vi "AddFailure_WithParent_ParentFailureIconSet.vi"() -> (0 "error out":errorcluster)   [LabVIEW 2017, in "ResultTreeListenerTest.lvlib"]
uses:
  ResultTreeListenerTest.lvlib
  ResultTreeListener/ResultTreeListener.lvclass
  ResultTree/ResultTree.lvclass
  Support/FakeTestCase/FakeTestCase.lvclass
  C:/Users/de200256/Code/neuperger/lvunit/Test/Test.lvclass
  275d98eb-69a7-4435-8809-2af3ffd1cf1d.vi
  ResultTree/Icon.ctl
  Support/FakeTestSuite/FakeTestSuite.lvclass
  C:/Users/de200256/Code/neuperger/lvunit/TestSuite/TestSuite.lvclass
panel:
  in  "Tree":string(tree)
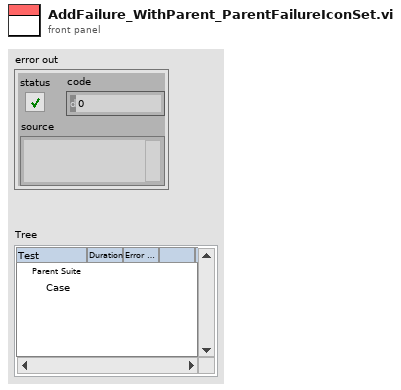
[diagram p1: front panel]
types:
  T1 = typedef "ResultTree.lvclass/Icon.ctl" = enum16{"None", "Passed", "Failed", "Error"}
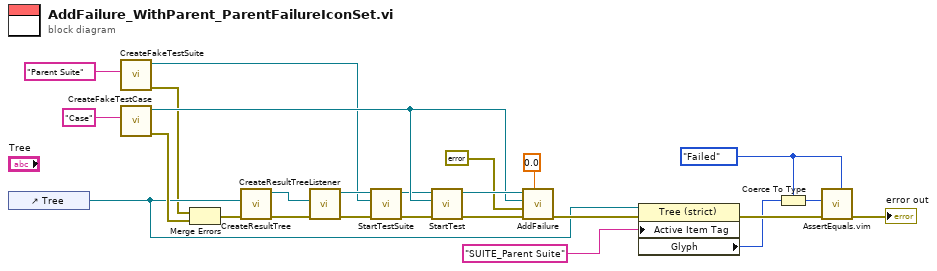
[diagram p0: block diagram]
diagram:
  w8 = Icon."Failed" ("Active Cell:String")
  n1 = control-ref of="Tree"() -> (w13:refnum<vi>)
  n2 = call "CreateFakeTestSuite.vi"("Name"="Parent Suite") -> ("error out"=w5:errorcluster, "FakeTestSuite out"=w1:refnum<class "FakeTestSuite.lvclass">)  [unwired: 9 in]
  n3 = call "CreateFakeTestCase.vi"("Name"="Case") -> ("error out"=w18:errorcluster, "FakeTestCase out"=w16:refnum<class "FakeTestCase.lvclass">)  [unwired: 9 in]
  n4 = Merge Errors(w5, w18) -> (w6:errorcluster)
  n5 = call "CreateResultTree.vi"("error in (no error)"=w6, "Tree Refnum"=w13) -> ("error out"=w25:errorcluster, "ResultTree out"=w24:refnum<class "ResultTree.lvclass">)  [unwired: 8 in]
  n6 = call "CreateResultTreeListener.vi"("error in (no error)"=w25, "ResultTree"=w24) -> ("error out"=w23:errorcluster, "ResultTreeListener out"=w3:refnum<class "ResultTreeListener.lvclass">)  [unwired: 8 in]
  n7 = call-dynamic "StartTestSuite.vi"("error in (no error)"=w23, "TestSuite"=w1, "ResultTreeListener in"=w3) -> ("error out"=w4:errorcluster, "ResultTreeListener out"=w2:refnum<class "ResultTreeListener.lvclass">)  [unwired: 7 in]
  n8 = call-dynamic "StartTest.vi"("error in (no error)"=w4, "Test"=w16, "ResultTreeListener in"=w2) -> ("error out"=w20:errorcluster, "ResultTreeListener out"=w19:refnum<class "ResultTreeListener.lvclass">)  [unwired: 7 in]
  n9 = call-dynamic "AddFailure.vi"("Time"=0.0, "error in (no error)"=w20, "Failure"=errorcluster {"status"=FALSE, "code"=0, "source"=""}, "Test"=w16, "ResultTreeListener in"=w19) -> ("error out"=w17:errorcluster)  [unwired: 5 in, 1 out]
  n10 = property class="Tree (strict)"(reference=w13, error in=w17, "Active Item Tag"="SUITE_Parent Suite" ("Active Item:Tag")) -> (error out=w14:errorcluster, "Glyph"=w11:i32)  [unwired: 1 out]
  n11 = Coerce To Type(0:w11, 1:w8) -> (2:w9:T1)
  n12 = call "AssertEquals.vim"("Expected"=w8, "error in (no error)"=w14, "Actual"=w9) -> ("error out"=→"error out":errorcluster)  [unwired: 8 in]
